vi "N sample current tasdk.vi"() -> ()   [LabVIEW 2020]
uses:
  <vilib>/DAQmx/read.llb/DAQmx Read (Analog 2D DBL NChan NSamp).vi
  <vilib>/DAQmx/miscellaneous.llb/DAQmx Fill In Error Info.vi
panel:
  out "Waveform Graph":dbl[][](graph)
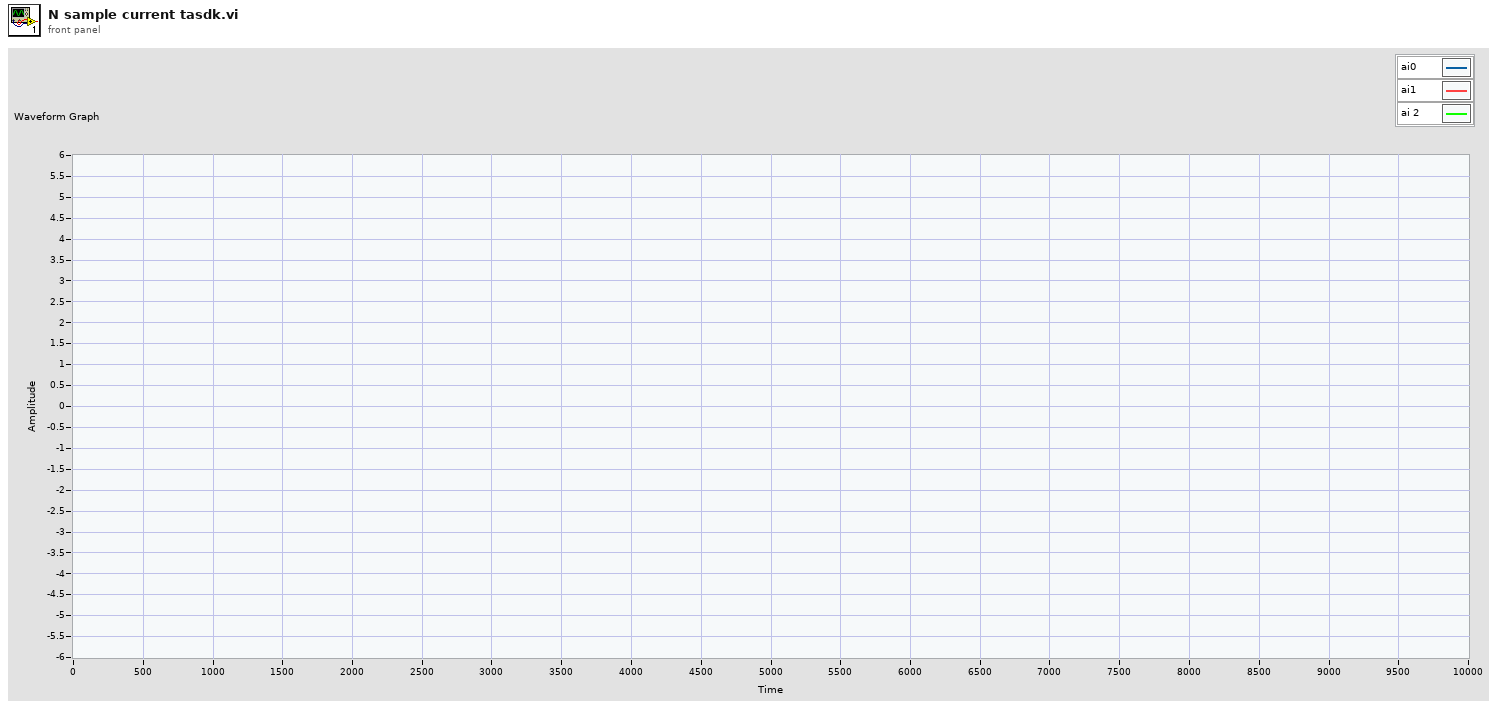
[diagram p1: front panel]
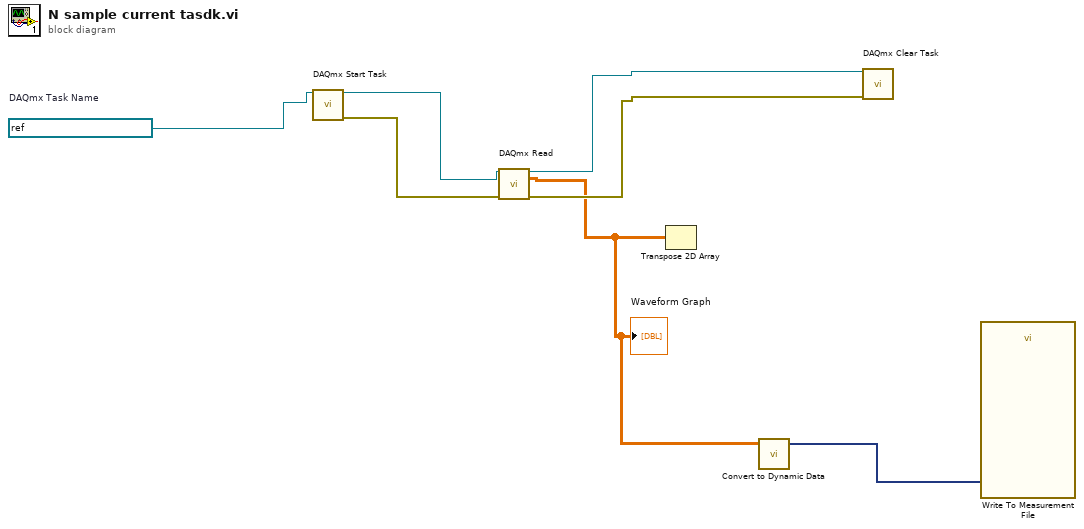
[diagram p0: block diagram]
diagram:
  w3 = refnum<k21> "N sample CurrentTask"  # DAQmx Task Name
  n1 = call <vilib>:"DAQmx Start Task.vi"("task/channels in"=w3) -> ("task out"=w7:refnum<k21>, "error out"=w4:errorcluster)  [unwired: 13 in]
  n2 = call-poly <vilib>:"DAQmx Read.vi"("task/channels in"=w7, "error in"=w4) -> ("task out"=w6:refnum<k21>, "data"=w1:dbl[][], "error out"=w5:errorcluster)  [unwired: 11 in]
  "Waveform Graph" <- w1
  n3 = Transpose 2D Array(2D array=w1) -> ()  [unwired: 1 out]
  n4 = call "Convert to Dynamic Data"("2D Array"=w1) -> ("Dynamic Data Type"=w2:dynamicdata)  [unwired: 3 in]
  n5 = call <vilib>:"DAQmx Clear Task.vi"("task in"=w6, "error in"=w5) -> ()  [unwired: 13 in, 1 out]
  n6 = call "Write To Measurement File"("Signals"=w2) -> ()  [unwired: 16 in, 3 out]
